vi "Continuous_Data_Packet_Receiver.vi"(8 "error in (no error)":errorcluster, 11 "COM Port":refnum<visa-resource-name>) -> (0 "error out":errorcluster, 1 "Processed bytes":u8[](array[numeric]), 2 "Raw Bytes":u8[](array[numeric]), 3 "Data Packet Statistics":T1, 5 "All Data Packet Statistics":T1[](array[typedef]))   [LabVIEW 2017]
uses:
  Controls/ADCP_UI/ADCP_UI_Data_Packet_Receiver_Parameters.ctl
  <vilib>/Instr/_visa.llb/VISA Flush IO Buffer Mask.ctl
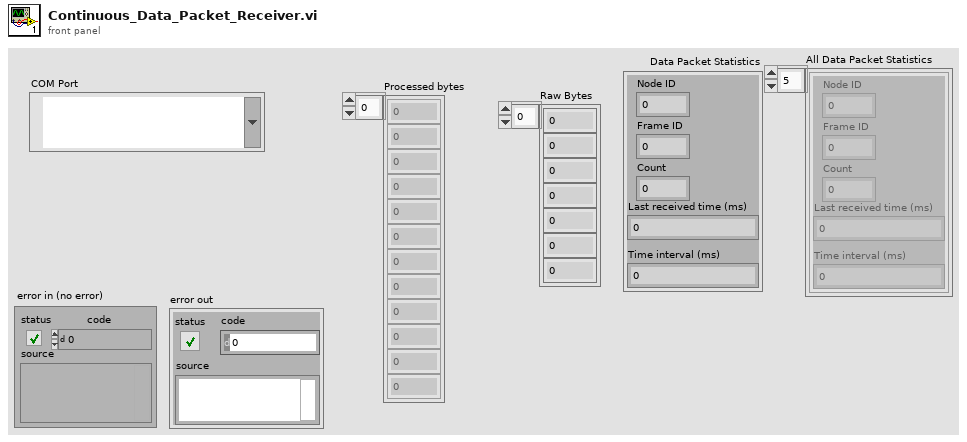
[diagram p1: front panel]
types:
  T1 = typedef "ADCP_UI_Data_Packet_Receiver_Parameters.ctl" = cluster{"Node ID":u32, "Frame ID":u32, "Count":u32, "Last received time (ms)":u32, "Time interval (ms)":u32}
  T2 = typedef "VISA Flush IO Buffer Mask.ctl" = u16
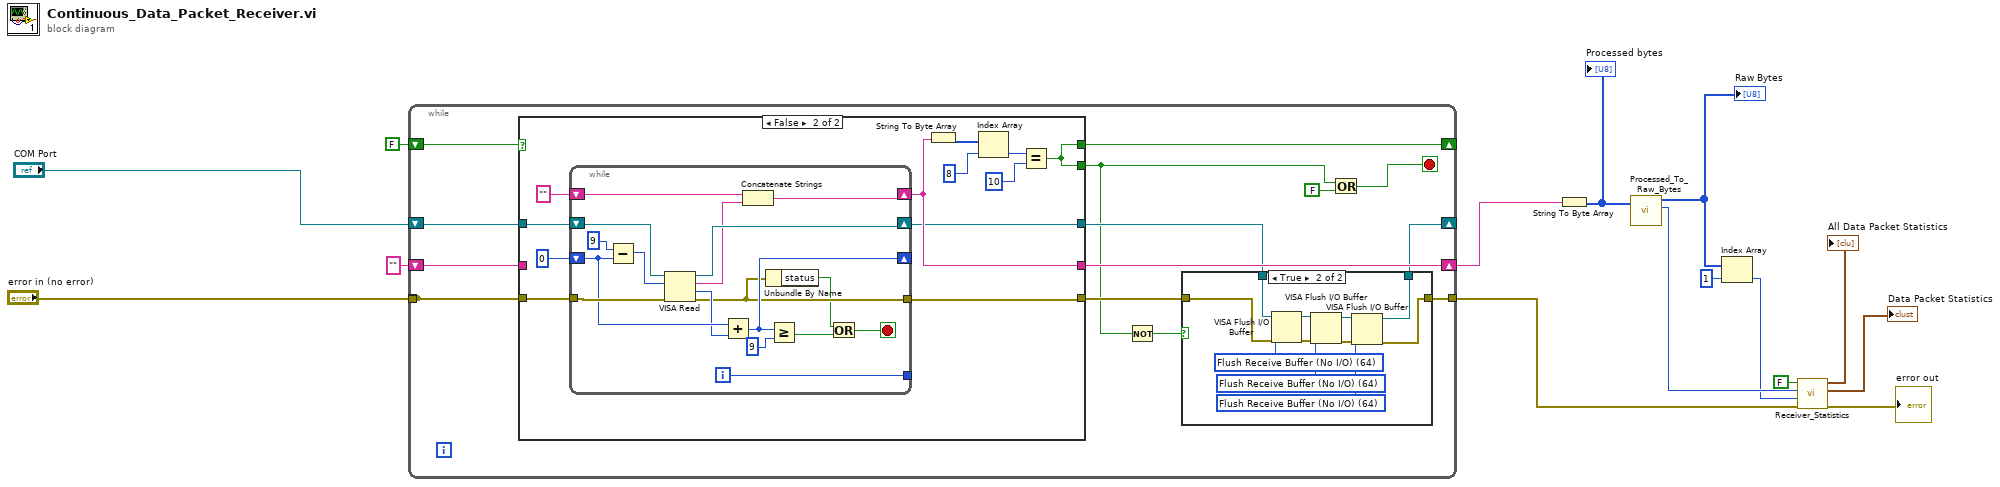
[diagram p0: block diagram]
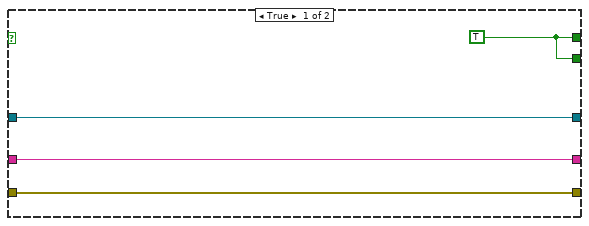
[diagram p3: hidden frame]
diagram:
  n1 = while {
    tunnel: "error in (no error)" -> [w24]
    shift-right: [w27] -> _
    shift-left: FALSE -> [w28]
    tunnel: [w22] -> w7
    shift-right: [w26] -> w12
    shift-left: "" -> [w25]
    shift-right: [w20] -> _
    shift-left: "COM Port" -> [w29]
    tunnel: [w24] -> _
    stop <- w19 stop-if-true
    n2 = case shown="False" w28 {
      tunnel: w24 -> [w45 w58]
      tunnel: w29 -> [w43 w56]
      tunnel: [w46 w50] -> w17
      tunnel: [w46 w50] -> w27
      tunnel: [w45 w49] -> w23
      tunnel: [w44 w48] -> w26
      tunnel: w25 -> [w44 _]
      tunnel: [w43 w47] -> w21
      frame True {
        w46 = TRUE
      }
      frame False {
        n3 = while {
          tunnel: w58 -> [w75]
          shift-right: [w65] -> _
          shift-left: 0 -> [w68]
          shift-right: [w71] -> w47
          shift-left: w56 -> [w72]
          shift-right: [w64] -> w48
          shift-left: "" -> [w70]
          tunnel: [w60] -> w49
          tunnel: [w63] -> _
          i -> [w63]
          stop <- w62 stop-if-true
          n4 = Subtract(x=9, y=w68) -> (x-y=w73:u32)
          n5 = VISA Read(VISA resource name=w72, byte count=w73, error in (no error)=w75) -> (VISA resource name out=w71:refnum<visa-resource-name>, read buffer=w69:string, return count=w67:u32, error out=w60:errorcluster)
          n6 = Add(x=w68, y=w67) -> (x+y=w65:u32)
          n7 = Concatenate Strings(w70, w69) -> (w64:string)
          n8 = Unbundle By Name(w60) -> ("status"=w59:bool)
          n9 = Greater Or Equal?(x=w65, y=u32 9) -> (x >= y?=w61:bool)
          n10 = Or(x=w59, y=w61) -> (x .or. y?=w62:bool)
        }
        n11 = String To Byte Array(string=w48) -> (unsigned byte array=w54:u8[])
        n12 = Index Array(array=w54, index=8) -> (element=w52:u8)
        n13 = Equal?(x=w52, y=u8 10) -> (x = y?=w50:bool)
      }
    }
    n14 = Not(x=w17) -> (.not. x?=w16:bool)
    n15 = case shown="True" w16 {
      tunnel: w23 -> [w31 w42]
      tunnel: [w31 w39] -> w22
      tunnel: w21 -> [w30 w38]
      tunnel: [w30 w35] -> w20
      frame False {
      }
      frame True {
        w32 = T2 64 items=["Flush Receive Buffer"=16, "Write Transmit Buffer to Device"=32, "Flush Receive Buffer (No I/O)"=64, "Flush Transmit Buffer"=128] ("Mask")
        w33 = T2 64 items=["Flush Receive Buffer"=16, "Write Transmit Buffer to Device"=32, "Flush Receive Buffer (No I/O)"=64, "Flush Transmit Buffer"=128] ("Mask")
        w34 = T2 64 items=["Flush Receive Buffer"=16, "Write Transmit Buffer to Device"=32, "Flush Receive Buffer (No I/O)"=64, "Flush Transmit Buffer"=128] ("Mask")
        n16 = VISA Flush I/O Buffer(VISA resource name=w38, mask (16)=w34, error in (no error)=w42) -> (VISA resource name out=w37:refnum<visa-resource-name>, error out=w41:errorcluster)
        n17 = VISA Flush I/O Buffer(VISA resource name=w37, mask (16)=w33, error in (no error)=w41) -> (VISA resource name out=w36:refnum<visa-resource-name>, error out=w40:errorcluster)
        n18 = VISA Flush I/O Buffer(VISA resource name=w36, mask (16)=w32, error in (no error)=w40) -> (VISA resource name out=w35:refnum<visa-resource-name>, error out=w39:errorcluster)
      }
    }
    n19 = Or(x=w17, y=FALSE) -> (x .or. y?=w19:bool)
  }
  n20 = String To Byte Array(string=w12) -> (unsigned byte array=w11:u8[])
  "Processed bytes" <- w11
  n21 = call "Processed_To_Raw_Bytes.vi"("Processed Bytes"=w11) -> ("Node ID"=w6:u8, "Raw Bytes"=w10:u8[])  [unwired: 1 in, 3 out]
  "Raw Bytes" <- w10
  n22 = Index Array(array=w10, index=1) -> (element=w5:u8)
  n23 = call "Receiver_Statistics.vi"("error in (no error)"=w7, "Frame ID"=w5, "Node ID"=w6, "Initialize ?"=FALSE) -> ("error out"=→"error out":errorcluster, "Output"=→"Data Packet Statistics":T1, "Received Packet Data"=→"All Data Packet Statistics":T1[])  [unwired: 5 in]
